vi "vjoylabview.vi"() -> ()   [LabVIEW 2020]
uses:
  C:/Program Files/vJoy/x86/vJoyInterfaceWrap.dll
  Program Files/vJoy/x86/vJoyInterfaceWrap.dll
  <vilib>/MakerHub/LINX/Public/Peripherals/Analog/Analog Read N Chans.vi
  <vilib>/MakerHub/LINX/Private/Local IO/LinxAnalogRead.vi
  <vilib>/MakerHub/LINX/Public/Utilities/Check Channel.vi
  <vilib>/MakerHub/LINX/Public/Utilities/Open Serial.vi
  <vilib>/MakerHub/LINX/Private/Utilties/Generate Error.vi
  <vilib>/MakerHub/LINX/LMH-LINX.lvlib
panel:
  out "Voltages":dbl[](array[numeric])
  in  "Serial Port":refnum<visa-resource-name>="N/A"
  in  "Stop Button":bool
  out "GetVJDStatus":i32(ring) items=["VJD_STAT_OWN", "VJD_STAT_FREE", "VJD_STAT_BUSY", "VJD_STAT_MISS", "VJD_STAT_UNKN"]
  out "AcquireVJD":bool
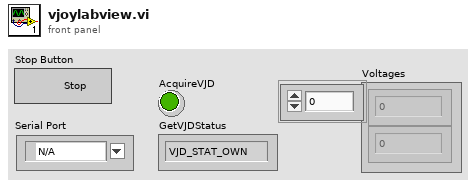
[diagram p1: front panel]
types:
  T1 = typedef "LMH-LINX.lvlib/LINX Ref.ctl" = cluster{"IO":T2, "Interface":T3, "LINX Device Config":T4}
  T2 = typedef "LMH-LINX.lvlib/Platform.ctl" = enum16{"Remote", "Local"}
  T3 = typedef "LMH-LINX.lvlib/Interface.ctl" = enum16{"Serial", "TCP"}
  T4 = typedef "LMH-LINX.lvlib/Device.lvlib/LINX Device Config.ctl" = cluster{"Interface":T3, "COM Port":refnum<visa-resource-name>, "TCP Configuration":T5, "Device Family":u8, "Device ID":u8, "Device Name":string, "TCP Ref":refnum<k5>, "Channels":T6}
  T5 = typedef "LMH-LINX.lvlib/Device.lvlib/TCP Config.ctl" = cluster{"IP Address":string, "Port":u16}
  T6 = typedef "LMH-LINX.lvlib/Channels.ctl" = cluster{"DI":u8[], "DO":u8[], "AI":u8[], "AO":u8[], "PWM":u8[], "QE":u8[], "UART":u8[], "I2C 2":u8[], "SPI":u8[], "CAN":u8[], "Servo":u8[], "AI Ref (V)":dbl, "AI Resolution (Bits)":u8, "AO Ref (V)":dbl, "AO Resolution (Bits)":u8}
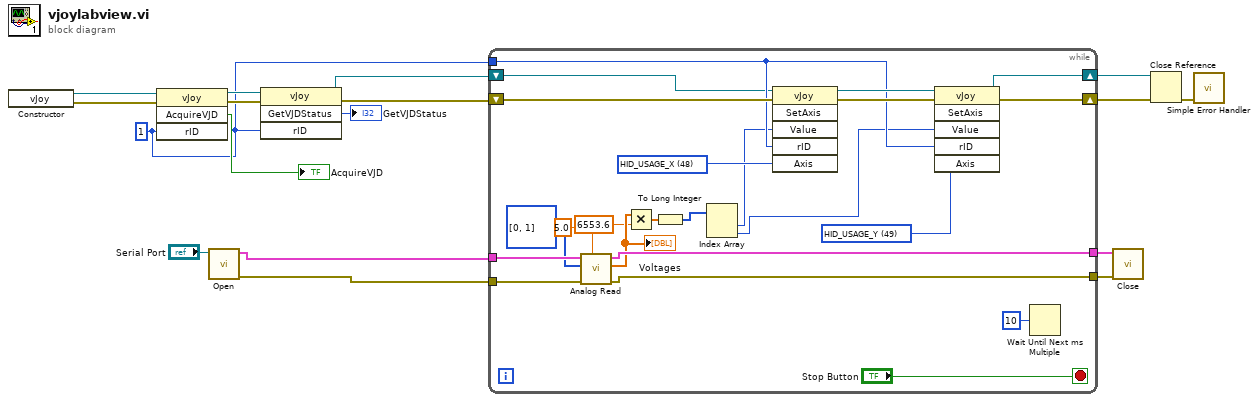
[diagram p0: block diagram]
diagram:
  w8 = u32 1 ("rID")
  n1 = constructor class="vJoy"() -> (reference out=w15:refnum<k24>, error out=w14:errorcluster)  [unwired: 3 in, 1 out]
  n2 = invoke class="vJoy" method="AcquireVJD"(reference=w15, error in=w14, "rID"=w8) -> (reference out=w13:refnum<k24>, error out=w12:errorcluster, "AcquireVJD"=→"AcquireVJD":bool)  [unwired: 1 in, 1 out]
  n3 = call-poly <vilib>:"Open.vi"("Serial Port"="Serial Port") -> ("Error Out"=w4:errorcluster, "LINX Resource"=w5:T1)  [unwired: 8 in, 1 out]
  n4 = invoke class="vJoy" method="GetVJDStatus"(reference=w13, error in=w12, "rID"=w8) -> (reference out=w11:refnum<k24>, error out=w10:errorcluster, "GetVJDStatus"=→"GetVJDStatus":i32)  [unwired: 1 in, 1 out]
  n5 = while {
    tunnel: w8 -> [w34]
    shift-right: [w39] -> w16
    shift-left: w11 -> [w18]
    shift-right: [w40] -> w17
    shift-left: w10 -> [w37]
    tunnel: w5 -> [w32]
    tunnel: w4 -> [w31]
    tunnel: [w30] -> w3
    tunnel: [w29] -> w2
    stop <- "Stop Button" stop-if-true
    w23 = 48 items=["HID_USAGE_X"=48, "HID_USAGE_Y"=49, "HID_USAGE_Z"=50, "HID_USAGE_RX"=51, "HID_USAGE_RY"=52, "HID_USAGE_RZ"=53, "HID_USAGE_SL0"=54, "HID_USAGE_SL1"=55, "HID_USAGE_WHL"=56, "HID_USAGE_POV"=57] ("Axis")
    w24 = 49 items=["HID_USAGE_X"=48, "HID_USAGE_Y"=49, "HID_USAGE_Z"=50, "HID_USAGE_RX"=51, "HID_USAGE_RY"=52, "HID_USAGE_RZ"=53, "HID_USAGE_SL0"=54, "HID_USAGE_SL1"=55, "HID_USAGE_WHL"=56, "HID_USAGE_POV"=57] ("Axis")
    n6 = call-poly <vilib>:"Analog Read.vi"("Analog Ref Override"=5.0, "Error In"=w31, "AI Channel(s)"=u8[] [0, 1], "LINX Resource"=w32) -> ("Error Out"=w29:errorcluster, "Voltages"=w28:dbl[], "LINX Resource"=w30:T1)  [unwired: 4 in, 1 out]
    "Voltages" <- w28
    n7 = Multiply(x=w28, y=6553.6) -> (x*y=w26:dbl[])
    n8 = To Long Integer(number=w26) -> (32bit integer=w22:i32[])
    n9 = Index Array(array=w22) -> (element #1=w21:i32, element #2=w20:i32)  [unwired: 2 in]
    n10 = invoke class="vJoy" method="SetAxis"(reference=w18, error in=w37, "Value"=w21, "rID"=w34, "Axis"=w23) -> (reference out=w36:refnum<k24>, error out=w35:errorcluster)  [unwired: 1 in, 4 out]
    n11 = invoke class="vJoy" method="SetAxis"(reference=w36, error in=w35, "Value"=w20, "rID"=w34, "Axis"=w24) -> (reference out=w39:refnum<k24>, error out=w40:errorcluster)  [unwired: 1 in, 4 out]
    n12 = Wait Until Next ms Multiple(millisecond multiple=u32 10) -> ()  [unwired: 1 out]
  }
  n13 = call <vilib>:"Close.vi"("Error In"=w2, "LINX Resource"=w3) -> ()  [unwired: 9 in, 1 out]
  n14 = Close Reference(reference=w16, error in (no error)=w17) -> (error out=w6:errorcluster)
  n15 = call <vilib>:"Simple Error Handler.vi"("error in (no error)"=w6) -> ()  [unwired: 4 in, 5 out]
